vi "_setPaneRef.vi"(7 "parentURL":string, 8 "error in (no error)":errorcluster, 9 "Name":string, 10 "Refnum":refnum<vi>, 11 "TagDB in":T1) -> (0 "error out":errorcluster, 2 "URL":string, 3 "TagDB out":T1)   [LabVIEW 2014, in "RefManager(dev).lvlib"]
uses:
  RefManager(dev).lvlib
  <userlib>/_NEVSTOP/TagDB/Core/tagDB_Def.ctl
  <userlib>/_NEVSTOP/TagDB/Core/_Support/Access/_setAnything.vi
  <userlib>/_NEVSTOP/TagDB/Core/_XNode/tagDB_setValue.xnode/tagDB_setValue.xnode
  <userlib>/_NEVSTOP/TagDB/Core/TagDB.lvlib
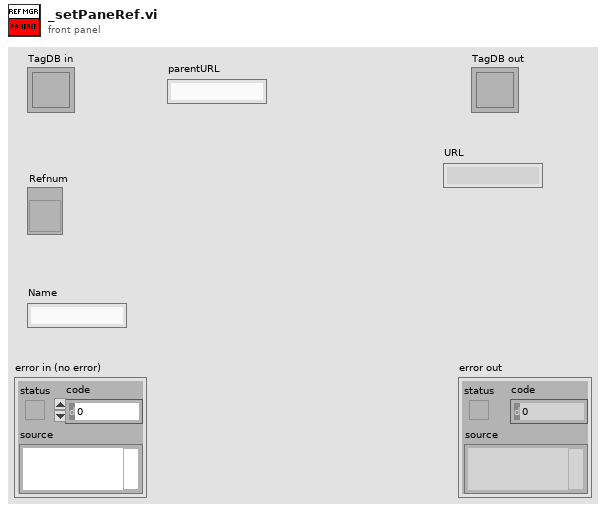
[diagram p1: front panel]
types:
  T1 = typedef "TagDB.lvlib/tagDB_Def.ctl" = refnum<k1>
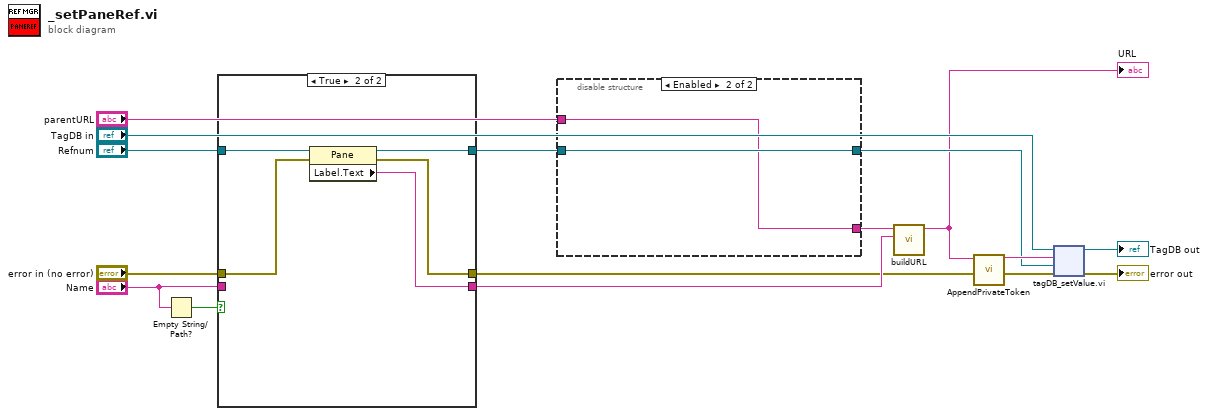
[diagram p0: block diagram]
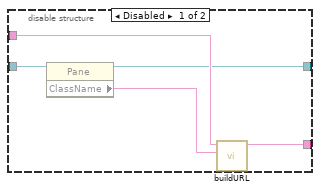
[diagram p2: hidden frame]
diagram:
  n1 = Empty String/Path?(string/path="Name") -> (empty?=w15:bool)
  n2 = case shown="True" w15 {
    tunnel: [w18 w21] -> w11
    tunnel: "Name" -> [w18 _]
    tunnel: "error in (no error)" -> [w17 w19]
    tunnel: [w17 w20] -> w6
    tunnel: "Refnum" -> [w16 w23]
    tunnel: [w16 w22] -> w4
    frame False {
    }
    frame True {
      n3 = property class="Pane"(reference=w23, error in=w19) -> (reference out=w22:refnum<vi>, error out=w20:errorcluster, "Label.Text"=w21:string)
    }
  }
  n4 = disable-structure shown="Enabled" {
    disable-tunnel: [w28 w29] -> w12
    disable-tunnel: "parentURL" -> [w27 w29]
    disable-tunnel: w4 -> [w26 w30]
    disable-tunnel: [w25 w30] -> w2
    frame Disabled {
      n5 = property class="Pane"(reference=w26) -> (reference out=w25:refnum<vi>, "ClassName"=w24:string)  [unwired: 1 in, 1 out]
      n6 = call <userlib>:"buildURL.vi"("DataName"=w24, "parentURL"=w27) -> ("DataURL"=w28:string)  [unwired: 9 in]
    }
    frame Enabled {
    }
  }
  n7 = call <userlib>:"buildURL.vi"("DataName"=w11, "parentURL"=w12) -> ("DataURL"=w1:string)  [unwired: 9 in]
  "URL" <- w1
  n8 = call <userlib>:"AppendPrivateToken.vi"("DataURL"=w1) -> ("String"=w3:string)  [unwired: 10 in]
  n9 = xnode "tagDB_setValue.vi"("DB Ref"="TagDB in", "name"=w3, "value"=w2, "Error In"=w6) -> ("DB Ref(dup)"=→"TagDB out":T1, "Error Out"=→"error out":errorcluster)  [unwired: 1 out]
